vi "FTW-Publisher-Publish.vi"(0 "FTW-Publisher In":refnum<class "FTW-Publisher.lvclass">, 5 "Header":string, 7 "Body":string, 11 "error in":errorcluster) -> (4 "FTW-Publisher Out":refnum<class "FTW-Publisher.lvclass">, 15 "error out":errorcluster)   [LabVIEW 2013, in "FTW-Publisher.lvclass"]
uses:
  FTW-Publisher.lvclass
  Package/Base/FTW-Message.lvclass
  FTW-Publisher.lvclass/FTW-Publisher.ctl
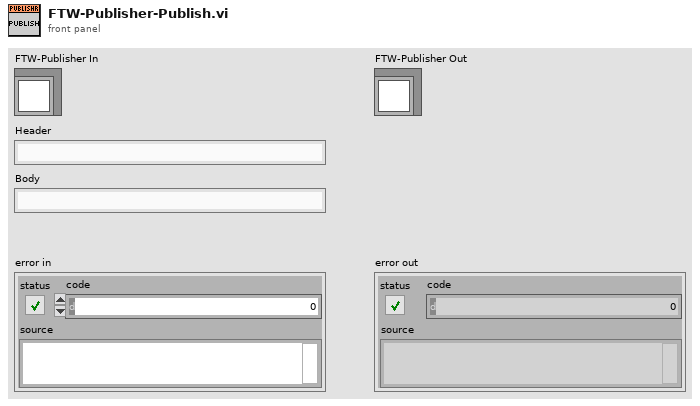
[diagram p1: front panel]
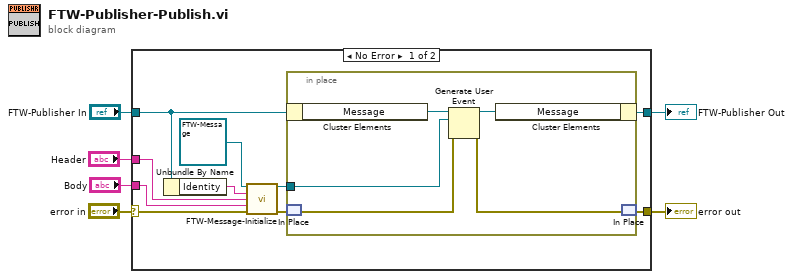
[diagram p0: block diagram]
diagram:
  n1 = case shown="No Error" "error in" {
    selector: "error in" -> [w15 w23]
    tunnel: [w14 w23] -> w3
    tunnel: [w16 w22] -> w5
    tunnel: "FTW-Publisher In" -> [w8 w22]
    tunnel: "Header" -> [w10 _]
    tunnel: "Body" -> [w9 _]
    frame No Error {
      n2 = Unbundle By Name(w8) -> ("Identity"=w7:string)
      n3 = call-dynamic "FTW-Message-Initialize.vi"("FTW Message"=refnum<class "FTW-Message.lvclass"> refnum, "Sender Identity"=w7, "Message Header"=w10, "Message Body"=w9, "error in"=w15) -> ("FTW Message out"=w12:refnum<class "FTW-Message.lvclass">, "error out"=w13:errorcluster)  [unwired: 9 in]
      n4 = in-place {
        in-place-border: w12 -> [w17]
        n5 = in-place-cluster #1(w8) -> ("Message"=w20:refnum<user-event>)
        n6 = in-place-match #2(w13) -> (w21:errorcluster)
        n7 = Generate User Event(user event=w20, event data cluster=w17, error in=w21) -> (user event out=w18:refnum<user-event>, error out=w19:errorcluster)  [unwired: 1 in]
        n8 = in-place-cluster #1("Message"=w18) -> (w16:refnum<class "FTW-Publisher.lvclass">)
        n9 = in-place-match #2(w19) -> (w14:errorcluster)
      }
    }
    frame Error {
    }
  }
  "FTW-Publisher Out" <- w5
  "error out" <- w3
